vi "NTV_Spare 2 Status.vi"(7 "Read(f) Write(t)":bool, 11 "Feeder State":T1) -> (3 "Feeder State Out":T1)   [LabVIEW 2023]
uses:
  TypeDefs/ENUM RB_Feeder State.ctl
  <vilib>/Rock Robotics/Network Tables/NT Read String.vi
  <vilib>/Rock Robotics/Network Tables/NT Write String.vi
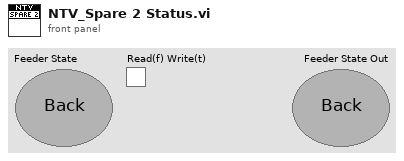
[diagram p1: front panel]
types:
  T1 = typedef "ENUM RB_Feeder State.ctl" = enum32{"Back", "Reversing", "Shooting"}
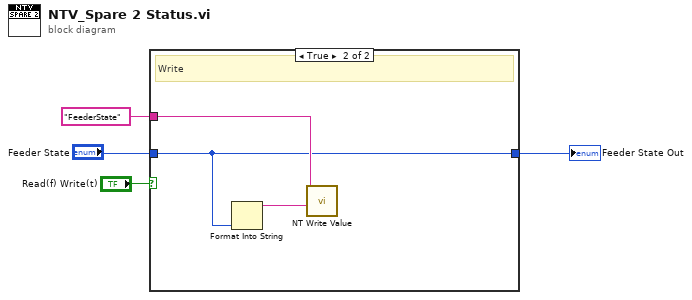
[diagram p0: block diagram]
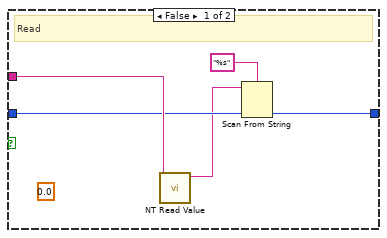
[diagram p2: hidden frame]
diagram:
  n1 = case shown="True" "Read(f) Write(t)" {
    tunnel: "Feeder State" -> [w8 w11]
    tunnel: "FeederState" ("Name") -> [w9 w12]
    tunnel: [w6 w11] -> w1
    frame False {
      (unwired) 0.0 ("Default Value")
      # "Read"
      n2 = call-poly <vilib>:"NT Read Value.vi"("name"=w9) -> ("value"=w7:string)  [unwired: 8 in, 2 out]
      n3 = Scan From String(format string="%s", input string=w7, default 1=w8) -> (output 1=w6:T1)  [unwired: 2 in, 3 out]
    }
    frame True {
      # "Write"
      n4 = Format Into String(w11) -> (resulting string=w10:string)  [unwired: 3 in, 1 out]
      n5 = call-poly <vilib>:"NT Write Value.vi"("value"=w10, "name"=w12) -> ()  [unwired: 9 in, 1 out]
    }
  }
  "Feeder State Out" <- w1
